vi "LV86_Flip.vi"(2 "Flip":enum16{"90¡", "180¡", "270¡"}(ring), 3 "Image":T1 {"Dialogs" format="%.0b"}) -> (1 "Image":T1 {"Dialogs" format="%.0b"})   [LabVIEW 2024]
doc: "This VI will flip the image by 90 degree imcrements clockwise"
uses:
  <userlib>/ImageProcessing/QTLIB_2595_LV86/QT_Image.ctl
panel:
  # "This VI will flip the image by 90 degree imcrements clockwise"
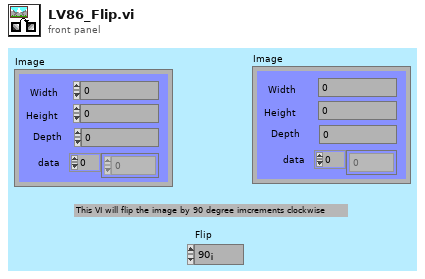
[diagram p1: front panel]
types:
  T1 = typedef "QT_Image.ctl" = cluster{"Width":i32, "Height":i32, "Depth":i32, "data":u8[], "Compressed data":u8[], "Color table":u32[], "Duration":i32, "Options":i32, "Timestamp":i32, "ID":i32, "Reserved":i32, "Dialogs":u32}
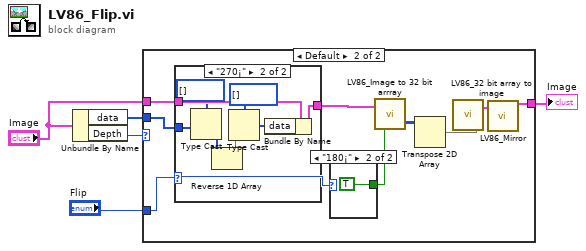
[diagram p0: block diagram]
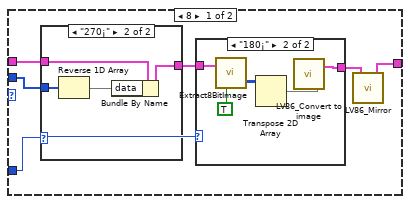
[diagram p2: hidden frame]
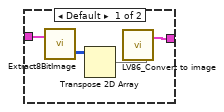
[diagram p4: hidden frame]
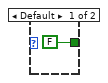
[diagram p5: hidden frame]
diagram:
  n1 = Unbundle By Name("Image") -> ("data"=w1:u8[], "Depth"=w5:i32)
  n2 = case shown="Default" w5 {
    tunnel: "Image" -> [w10 w33]
    tunnel: [w8 w31] -> w3
    tunnel: "Flip" -> [w7 w28]
    tunnel: w1 -> [w6 w26]
    frame 8 {
      n3 = case shown="\"270¡\"" w7 {
        tunnel: w6 -> [_ w16]
        tunnel: w10 -> [w12 w14]
        tunnel: [w12 w13] -> w9
        frame Default {
        }
        frame "270¡" {
          n4 = Reverse 1D Array(array=w16) -> (reversed array=w15:u8[])
          n5 = Bundle By Name(cluster=w14, "data"=w15) -> (w13:T1)
        }
      }
      n6 = case shown="\"180¡\"" w7 {
        tunnel: w9 -> [w20 w25]
        tunnel: [w17 w22] -> w11
        frame Default {
          n7 = call <userlib>:"Extract8BitImage.vi"("Image in"=w20) -> ("Intensity Graph"=w19:u8[][])  [unwired: 1 in, 1 out]
          n8 = Transpose 2D Array(2D array=w19) -> (transposed array=w18:u8[][])
          n9 = call <userlib>:"LV86_Convert to image.vi"("Intensity Graph"=w18) -> ("Image Out"=w17:T1)  [unwired: 2 in]
        }
        frame "180¡" {
          n10 = call <userlib>:"Extract8BitImage.vi"("Flip?"=TRUE, "Image in"=w25) -> ("Intensity Graph"=w24:u8[][])  [unwired: 1 out]
          n11 = Transpose 2D Array(2D array=w24) -> (transposed array=w23:u8[][])
          n12 = call <userlib>:"LV86_Convert to image.vi"("Intensity Graph"=w23) -> ("Image Out"=w22:T1)  [unwired: 2 in]
        }
      }
      n13 = call <userlib>:"LV86_Mirror.vi"("Image"=w11) -> ("Image"=w8:T1)  [unwired: 2 out]
    }
    frame Default {
      n14 = case shown="\"270¡\"" w28 {
        tunnel: w26 -> [_ w42]
        tunnel: w33 -> [w37 w45]
        tunnel: [w37 w44] -> w32
        frame Default {
        }
        frame "270¡" {
          n15 = Type Cast(type=u32[] [] ("Array Constant"), x=w42) -> (*(type *) &x=w41:u32[])
          n16 = Reverse 1D Array(array=w41) -> (reversed array=w40:u32[])
          n17 = Type Cast(type=u8[] [] ("Array Constant"), x=w40) -> (*(type *) &x=w38:u8[])
          n18 = Bundle By Name(cluster=w45, "data"=w38) -> (w44:T1)
        }
      }
      n19 = case shown="\"180¡\"" w28 {
        tunnel: [FALSE TRUE] -> w27
        frame Default {
        }
        frame "180¡" {
        }
      }
      n20 = call <userlib>:"LV86_Image to 32 bit arrray.vi"("Flip?"=w27, "Image In"=w32) -> ("Intensity Graph"=w30:u32[][])  [unwired: 1 out]
      n21 = Transpose 2D Array(2D array=w30) -> (transposed array=w29:u32[][])
      n22 = call <userlib>:"LV86_32 bit array to image.vi"("Intensity Graph"=w29) -> ("Image Out"=w34:T1)  [unwired: 2 in]
      n23 = call <userlib>:"LV86_Mirror.vi"("Image"=w34) -> ("Image"=w31:T1)  [unwired: 2 out]
    }
  }
  "Image" <- w3
